vi "MEASURE_hysteresis_multiple_SHG gate_pmt-final - Set voltage_1022D.vi"() -> ()   [LabVIEW 2020]
uses:
  <instrlib>/Keithley 24XX/Public/Data/Read (Multiple Points).vi
  <vilib>/Utility/file.llb/Write Delimited Spreadsheet (DBL).vi
  <instrlib>/Keithley 24XX/Keithley 24XX.lvlib
  <vilib>/Analysis/NI_AALBase.lvlib
panel:
  in  "B Reference Source":u8(ring) items=["External", "Internal", "Internal Sweep"]
  in  "Sample Time (0.01-100s)":u16(ring) items=["62.5 mHz", "125 mHz", "250 mHz", "500 mHz", "1 Hz", "2 Hz", "4 Hz", "8Hz", "16 Hz", "32 Hz", "64 Hz", "128 Hz", "256 Hz", "512 Hz", "Trigger "]
  in  "auto phase B":bool
  in  "B reference Manual Phase":dbl=0.05
  in  "B harmonic 2":u8
  in  "B harmonic 1":u8
  in  "B Sine Output Amplitude":dbl=0.05
  in  "B Input Connection":u16(ring) items=["Single-Ended Voltage", "Differential Voltage", "1 MOhm Current Gain", "100 MOhm Current Gain"]
  in  "B frequency":dbl=50.0 format="%#_13g"
  in  "A Reference Source":u8(ring) items=["External", "Internal", "Internal Sweep"]
  in  "Sample Time (0.01-100s)":u16(ring) items=["62.5 mHz", "125 mHz", "250 mHz", "500 mHz", "1 Hz", "2 Hz", "4 Hz", "8Hz", "16 Hz", "32 Hz", "64 Hz", "128 Hz", "256 Hz", "512 Hz", "Trigger "]
  in  "auto phase A":bool
  in  "A reference Manual Phase":dbl=0.05
  in  "A harmonic 2":u8
  in  "Channel A/B for Parameter1":u8(ring) items=["Channel A", "Channel B"]
  out "top gate leaking":dbl=2.469318360898143e-10
  in  "Parameter1":u16(ring)=1 items=["X", "Y", "R", "Theta", "Frequency", "Noise", "Xh1", "Yh1", "Rh1", "Theta h1", "Xh2", "Yh2", "Rh2", "Theta h2"]
  in  "A harmonic 1":u8
  in  "Set voltage (T)":bool=TRUE
  in  "back Vg final Value":dbl=6.0
  in  "Gate sequence":dbl
  out "while loop":dbl
  in  "bottom gate-off set":dbl=-5.0
  in  "0ff set{T}/no off set[F]":bool
  out "XY Graph 4":cluster{dbl[], sgl[]}(graph)
  out "XY Graph 3":cluster{dbl[], sgl[]}(graph)
  out "back gate leaking":dbl=2.469318360898143e-10
  out "top gate voltage":dbl format="%#_13g"
  in  "Compliance  Level (1uA)":dbl=1.9999999995789155e-07
  in  "Source Mode  (0: Voltage)":u16(ring) items=["Voltage", "Current"]
  in  "Serial Configuration":T1={"Baud Rate"=9600, "Parity"=0, "Data Bits"=8, "Stop Bits"=10, "Flow Control"=0} {"Flow Control" items=["None", "XON/XOFF", "RTS/CTS", "XON/XOFF & RTS/CTS", "DTR/DSR", "XON/XOFF & DTR/DSR"]; "Stop Bits" items=["1.0"=10, "1.5"=15, "2.0"=20]; "Data Bits" items=["7"=7, "8"=8]; "Parity" items=["None", "Odd", "Even", "Mark", "Space"]; "Baud Rate" items=["300"=300, "600"=600, "1200"=1200, "2400"=2400, "4800"=4800, "9600"=9600, "19200"=19200]}
  in  "back gate address":refnum<visa-resource-name>="GPIB0::25::INSTR"
  in  "top gate thickness":dbl=10.0
  in  "back gate thickness":dbl=30.0
  in  "pure field (T)/pure doping (F)":bool
  out "loop run":i32=2
  in  "loop #":i32=2
  in  "Save data or not":bool=TRUE
  in  "path (folder + filename)":string="C:\\Users\\User\\Data\\Jason\\03282019\\ pure_bottom_high_6v_rato3 with light2"
  in  "Clear Plot":bool
  out "LOCKIN Measurement1":dbl=0.9110010000000001
  out "back gate voltage":dbl format="%#_13g"
  in  "GATE STEP(mv)":i32=450
  in  "GATE Low Value (default 0)":dbl
  in  "GATE High Value":dbl=18.0
  in  "Function (0: Volts) 2":u16(ring) items=["Volts", "Current", "Resistance"]
  in  "Source Compaliance":dbl=1.000000000000001e-07
  in  "topgate address":refnum<visa-resource-name>="GPIB0::18::INSTR"
  in  "SD stabilization(S) 2":dbl=0.1 format="%#_13g"
  in  "A Sine Output Amplitude":dbl=0.05
  in  "GATE / SD stablization 3":dbl=0.1 format="%#_13g"
  in  "A Sine output frequency":dbl=50.0 format="%#_13g"
  in  "A Input Connection":u16(ring) items=["Single-Ended Voltage", "Differential Voltage", "1 MOhm Current Gain", "100 MOhm Current Gain"]
  in  "LOCKIN address":refnum<visa-resource-name>="GPIB0::8::INSTR"
  # "Gate2400(Back) Setting"
  # "Lock-in"
  # "Channel A"
  # "Gate2400(Top) Setting"
  # "Channel B"
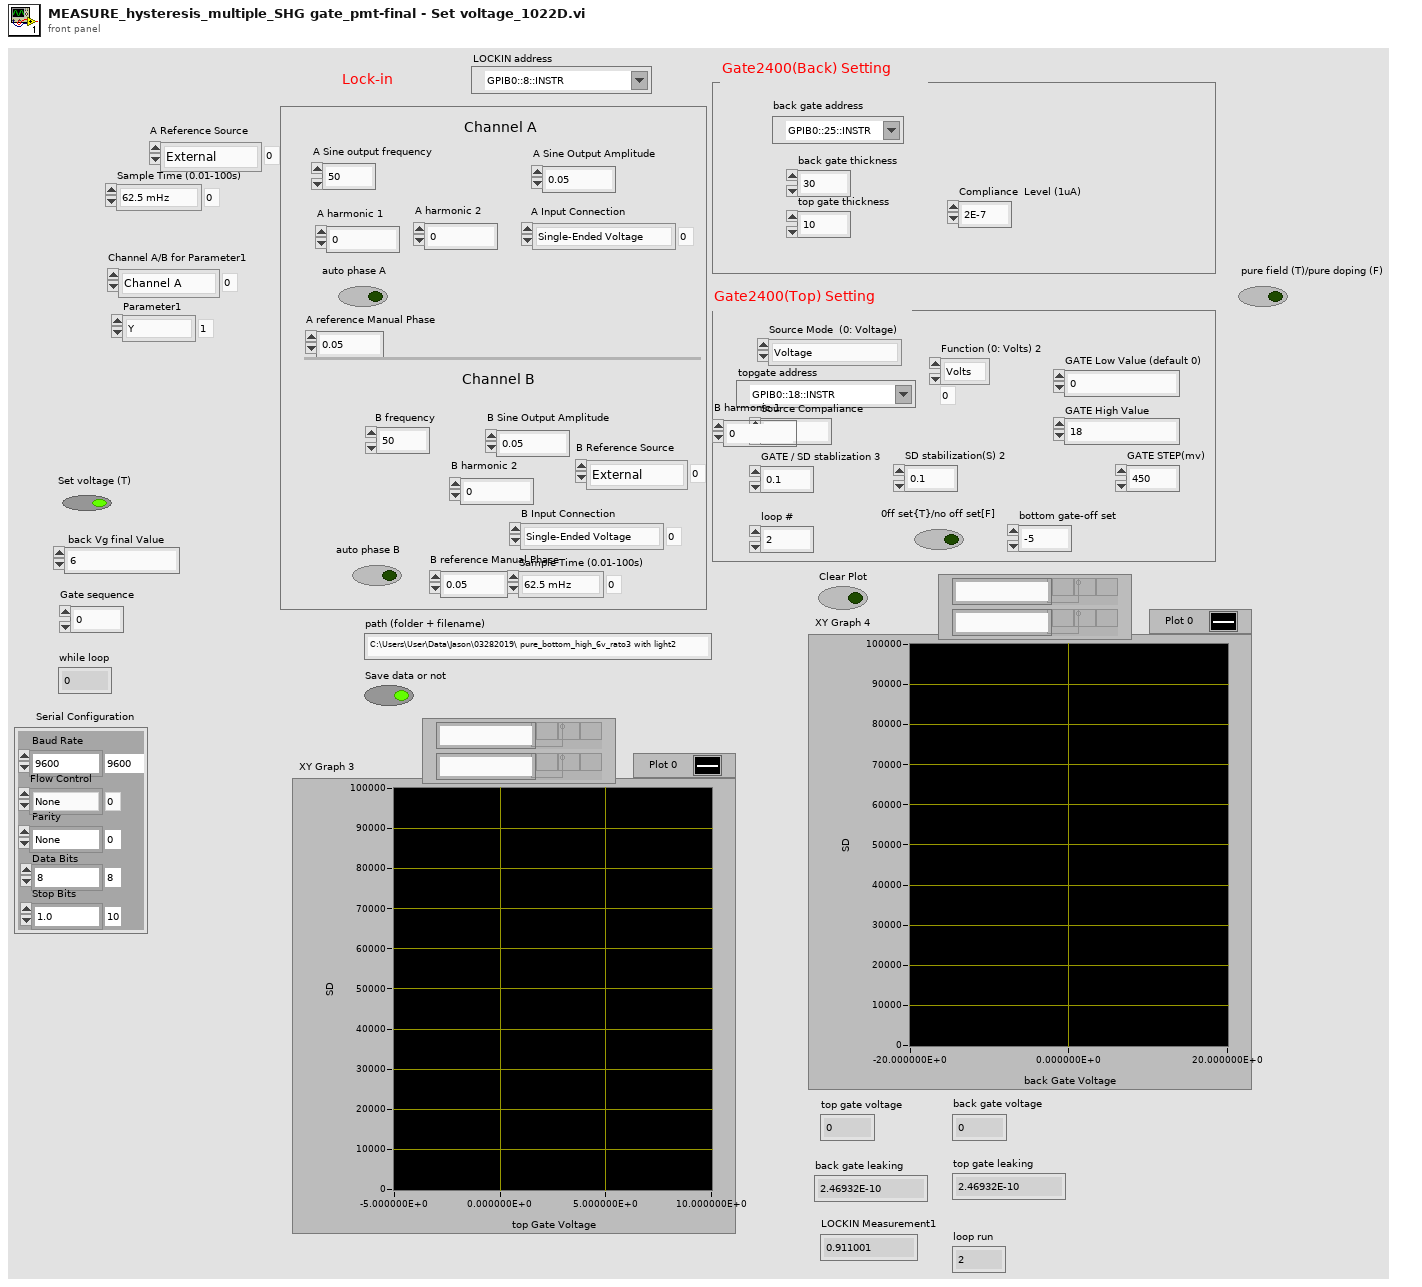
[diagram p1: front panel]
types:
  T1 = cluster{"Baud Rate":u32, "Parity":u16, "Data Bits":u16, "Stop Bits":u16, "Flow Control":u16}
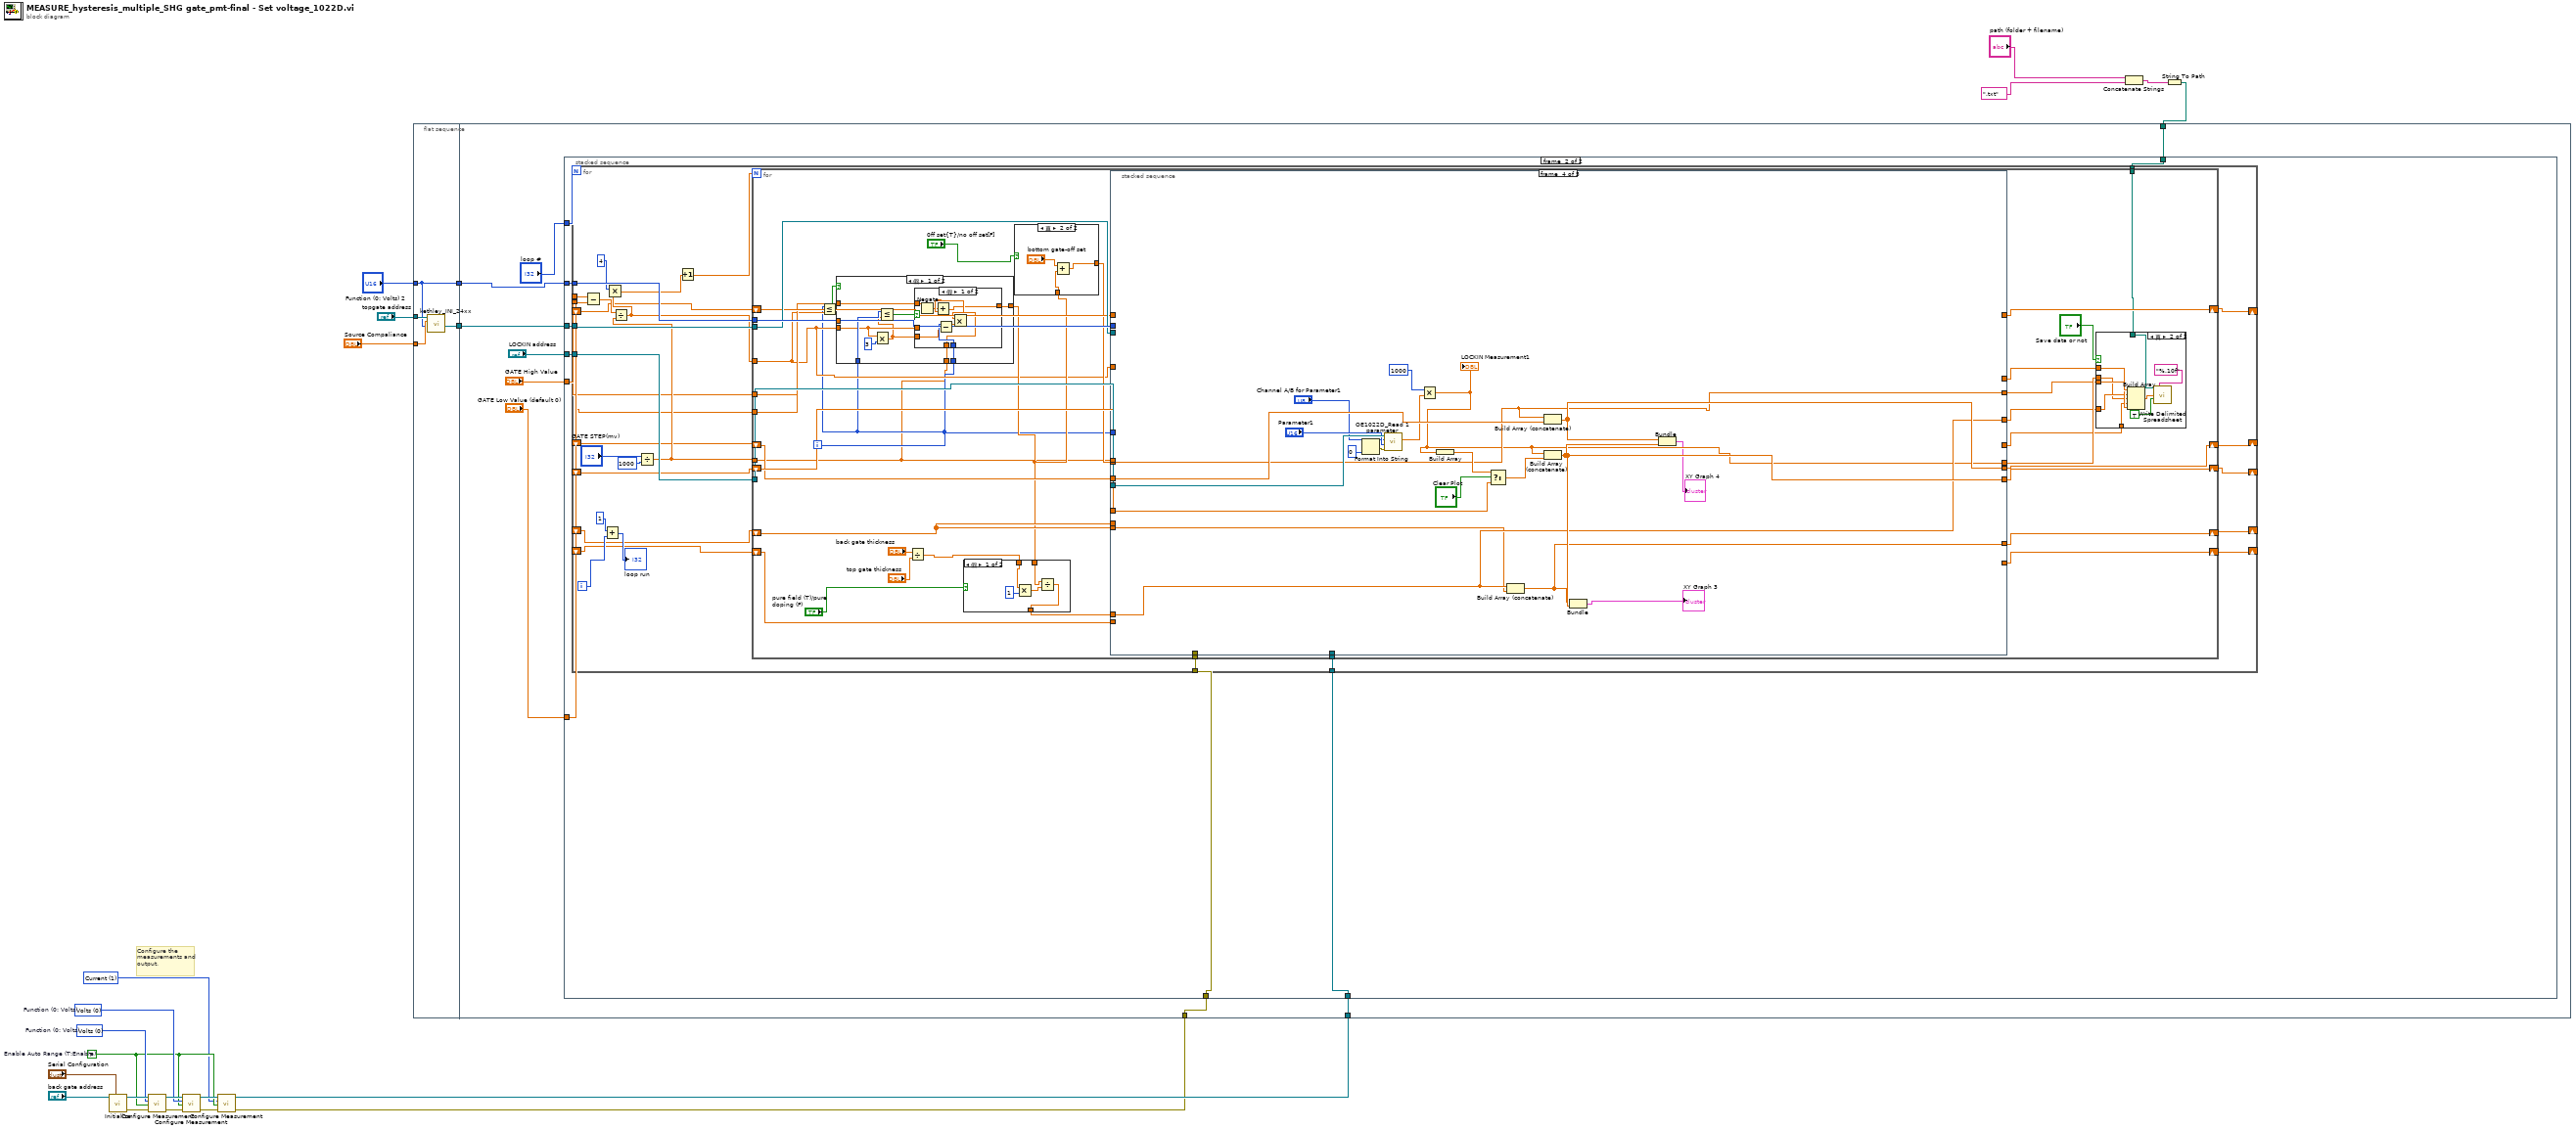
[diagram p0: block diagram]
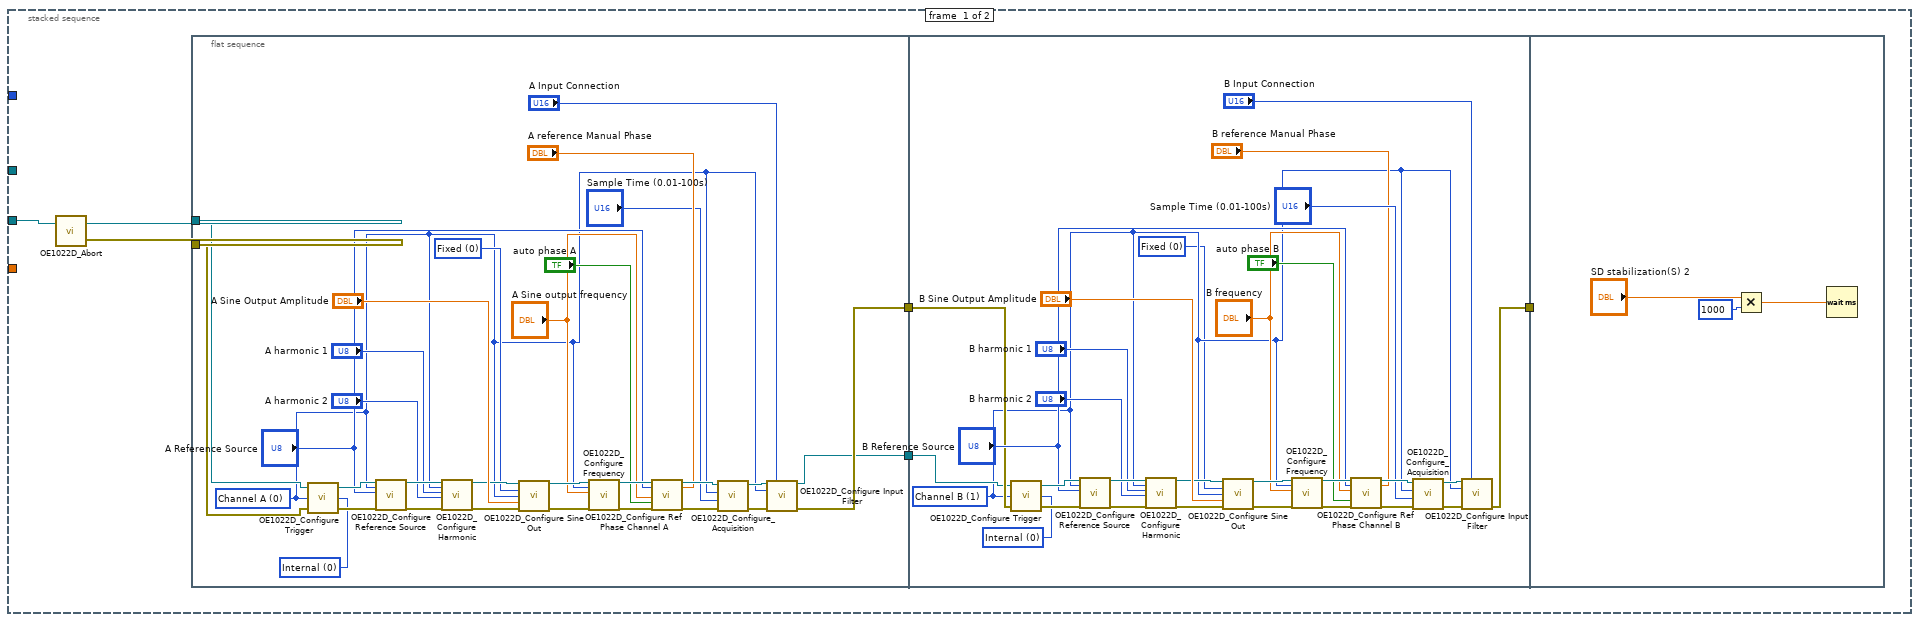
[diagram p2: hidden frame]
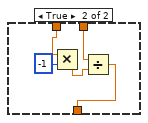
[diagram p4: hidden frame]
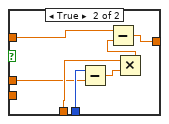
[diagram p6: hidden frame]
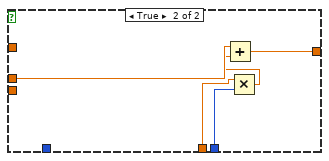
[diagram p7: hidden frame]
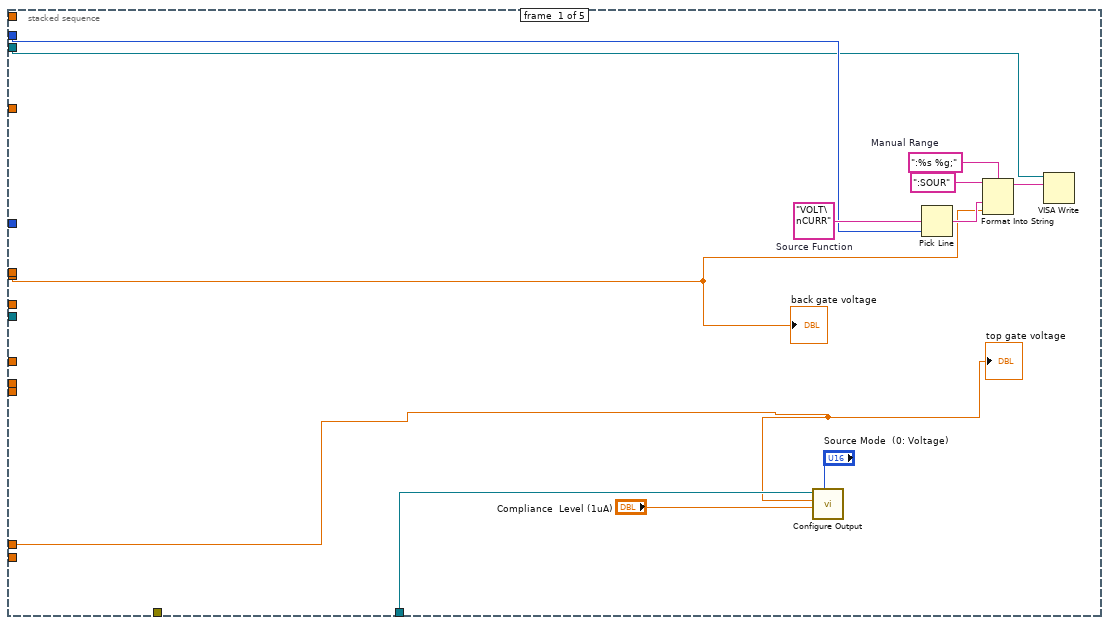
[diagram p8: hidden frame]
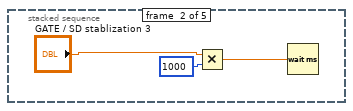
[diagram p9: hidden frame]
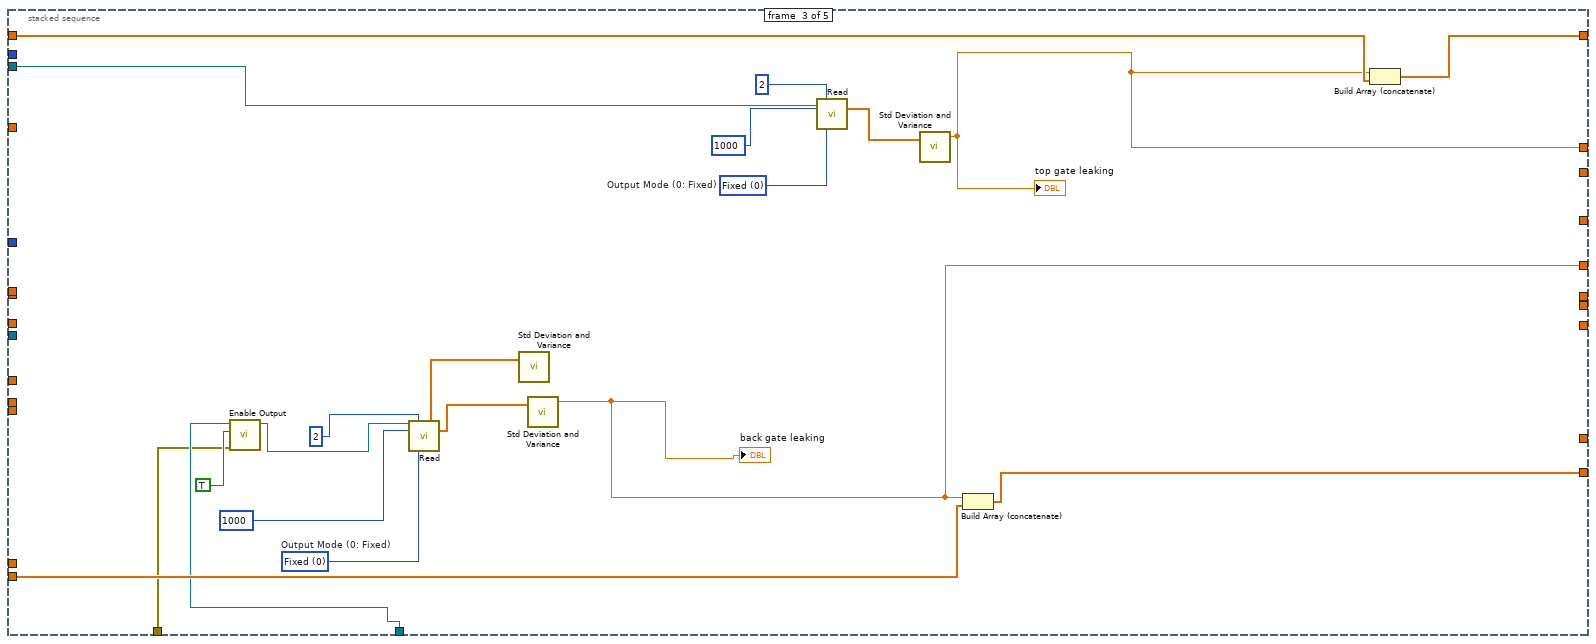
[diagram p10: hidden frame]
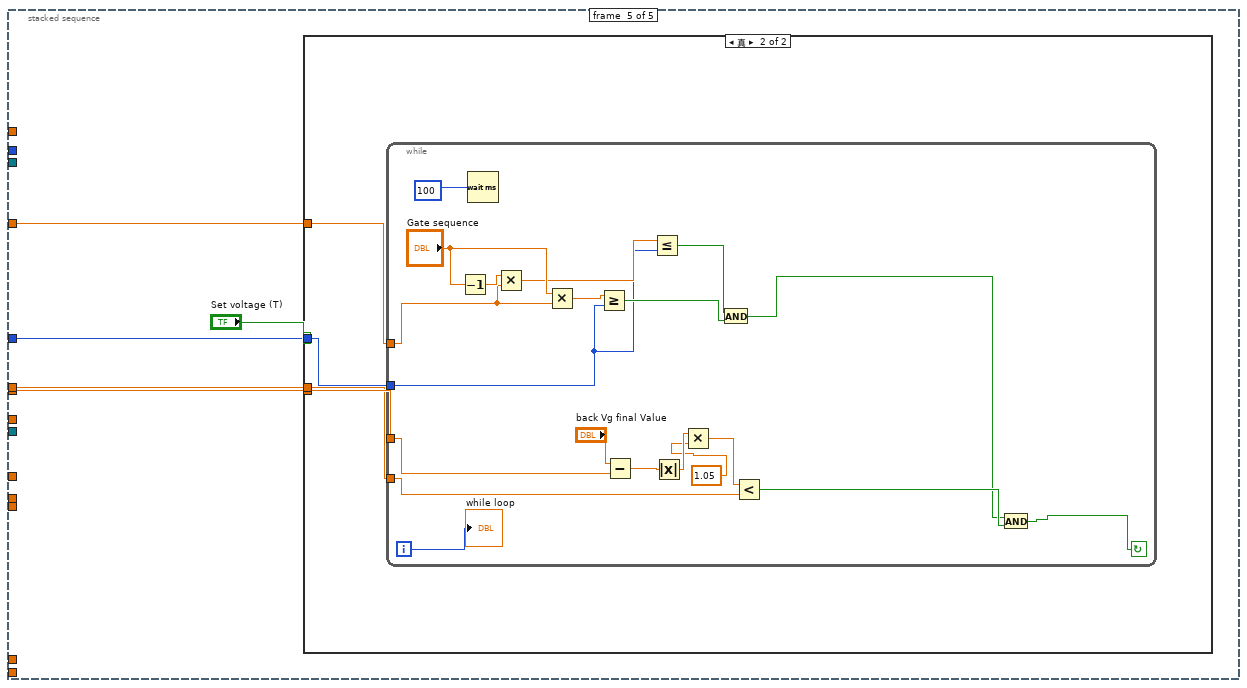
[diagram p11: hidden frame]
diagram:
  w3 = u16 1 items=["Volts", "Current", "Resistance"] ("Function (0: Volts)")
  w4 = TRUE  # Enable Auto Range (T:Enable)
  w7 = u16 0 items=["Volts", "Current", "Resistance"]  # Function (0: Volts)
  w8 = u16 0 items=["Volts", "Current", "Resistance"]  # Function (0: Volts)
  # "Configure the measurements and output."
  n1 = call <instrlib>:"Initialize.vi"("Serial Configuration"="Serial Configuration", "VISA resource name"="back gate address") -> ("error out"=w13:errorcluster, "VISA resource name out"=w14:refnum<visa-resource-name>)  [unwired: 8 in]
  n2 = call <instrlib>:"Configure Measurement.vi"("error in (no error)"=w13, "Enable Auto Range (T:Enable)"=w4, "Function (0: Volts)"=w8, "VISA resource name"=w14) -> ("error out"=w12:errorcluster, "VISA resource name out"=w11:refnum<visa-resource-name>)  [unwired: 6 in]
  n3 = call <instrlib>:"Configure Measurement.vi"("error in (no error)"=w12, "Enable Auto Range (T:Enable)"=w4, "Function (0: Volts)"=w7, "VISA resource name"=w11) -> ("error out"=w5:errorcluster, "VISA resource name out"=w6:refnum<visa-resource-name>)  [unwired: 6 in]
  n4 = call <instrlib>:"Configure Measurement.vi"("error in (no error)"=w5, "Enable Auto Range (T:Enable)"=w4, "Function (0: Volts)"=w3, "VISA resource name"=w6) -> ("error out"=w1:errorcluster, "VISA resource name out"=w2:refnum<visa-resource-name>)  [unwired: 6 in]
  n5 = flat-sequence {
    tunnel: "topgate address" -> [w27]
    tunnel: "Source Compaliance" -> [w26]
    tunnel: "Function (0: Volts) 2" -> [w24]
    tunnel: [w25] -> w20
    tunnel: [w24] -> w19
    tunnel: w20 -> [w35]
    tunnel: w19 -> [w34]
    tunnel: w15 -> [w31]
    tunnel: w2 -> [w29]
    tunnel: w1 -> [w28]
    frame #0 {
      n6 = call "kethley_INI_24xx.vi"("Function (0: Volts) in"=w24, "Source Compaliance"=w26, "VISA Return in"=w27) -> ("VISA resource name out"=w25:refnum<visa-resource-name>)  [unwired: 8 in]
    }
    frame #1 {
      n7 = stacked-sequence {
        tunnel: "LOCKIN address" -> [w42 w111]
        tunnel: w35 -> [_ w112]
        tunnel: w34 -> [_ w113]
        tunnel: "GATE High Value" -> [_ w109]
        tunnel: "GATE Low Value (default 0)" -> [_ w110]
        tunnel: w31 -> [_ w108]
        tunnel: "loop #" -> [_ w107]
        tunnel: w29 -> [_ w106]
        tunnel: w28 -> [_ w105]
        frame #0 {
          n8 = call <instrlib>:"OE1022D_Abort.vi"("VISA resource name"=w42) -> ("error out"=w40:errorcluster, "VISA resource name out"=w41:refnum<visa-resource-name>)  [unwired: 1 in]
          n9 = flat-sequence {
            tunnel: w41 -> [w72]
            tunnel: [w60] -> w39
            tunnel: w40 -> [w71]
            tunnel: [w45] -> w37
            tunnel: w39 -> [w79]
            tunnel: [w78] -> w38
            tunnel: w37 -> [w77]
            tunnel: w38 -> [_]
            frame #0 {
              w44 = u8 0 items=["Fixed", "Linear", "Log"] ("SineOut Mode")
              w46 = u16 0 items=["Internal", "External"] ("Trigger Source (0: Internal)")
              w43 = u8 0 items=["Channel A", "Channel B"] ("OE1022D A/B")
              n10 = call <instrlib>:"OE1022D_Configure Trigger.vi"("Trigger Source (0: Internal)"=w46, "error in (no error)   2"=w71, "OE1022D A/B"=w43, "VISA resource name   2"=w72) -> ("error out   2"=w65:errorcluster, "VISA resource name out   2"=w66:refnum<visa-resource-name>)
              n11 = call <instrlib>:"OE1022D_Configure Reference Source.vi"("VISA resource name"=w66, "OE1022D A/B"=w43, "Reference Source"="A Reference Source", "error in (no error)"=w65) -> ("VISA resource name out"=w64:refnum<visa-resource-name>, "error out"=w62:errorcluster)  [unwired: 14 in]
              n12 = call <instrlib>:"OE1022D_Configure Harmonic.vi"("VISA resource name"=w64, "OE1022D A/B"=w43, "Harmonic 1"="A harmonic 1", "Harmonic 2"="A harmonic 2", "error in (no error)"=w62) -> ("VISA resource name out"=w63:refnum<visa-resource-name>, "error out"=w61:errorcluster)  [unwired: 13 in]
              n13 = call <instrlib>:"OE1022D_Configure Sine Out.vi"("VISA resource name"=w63, "SineOut Mode"=w44, "OE1022D A/B"=w43, "Sine Output Amplitude (V)"="A Sine Output Amplitude", "error in (no error)"=w61) -> ("VISA resource name out"=w69:refnum<visa-resource-name>, "error out"=w68:errorcluster)  [unwired: 9 in]
              n14 = call <instrlib>:"OE1022D_Configure Frequency.vi"("VISA resource name"=w69, "OE1022D A/B"=w43, "Internal Frequency(Hz)"="A Sine output frequency", "error in (no error)"=w68) -> ("VISA resource name out"=w59:refnum<visa-resource-name>, "error out"=w54:errorcluster)  [unwired: 14 in]
              n15 = call <instrlib>:"OE1022D_Configure Ref Phase Channel A.vi"("VISA resource name"=w59, "Reference Source"="A Reference Source", "Internal Frequency(Hz)"="A Sine output frequency", "Auto Phase (T: Enabled)"="auto phase A", "error in (no error)"=w54, "Manual Phase  (degree)"="A reference Manual Phase") -> ("VISA resource name out"=w58:refnum<visa-resource-name>, "error out"=w55:errorcluster)  [unwired: 12 in]
              n16 = call <instrlib>:"OE1022D_Configure_Acquisition.vi"("VISA resource name"=w58, "Channel A/B"=w43, "Sample time (s)"="Sample Time (0.01-100s)", "error in (no error)"=w55) -> ("VISA resource name out"=w57:refnum<visa-resource-name>, "error out"=w56:errorcluster)  [unwired: 5 in]
              n17 = call <instrlib>:"OE1022D_Configure Input Filter.vi"("VISA resource name"=w57, "Input Source"="A Input Connection", "OE1022D A/B"=w43, "error in (no error)"=w56) -> ("VISA resource name out"=w45:refnum<visa-resource-name>, "error out"=w60:errorcluster)  [unwired: 10 in]
            }
            frame #1 {
              w73 = u8 0 items=["Fixed", "Linear", "Log"] ("SineOut Mode")
              w80 = u16 0 items=["Internal", "External"] ("Trigger Source (0: Internal)")
              w74 = u8 1 items=["Channel A", "Channel B"] ("OE1022D A/B")
              n18 = call <instrlib>:"OE1022D_Configure Trigger.vi"("Trigger Source (0: Internal)"=w80, "error in (no error)   2"=w79, "OE1022D A/B"=w74, "VISA resource name   2"=w77) -> ("error out   2"=w96:errorcluster, "VISA resource name out   2"=w97:refnum<visa-resource-name>)
              n19 = call <instrlib>:"OE1022D_Configure Reference Source.vi"("VISA resource name"=w97, "OE1022D A/B"=w74, "Reference Source"="B Reference Source", "error in (no error)"=w96) -> ("VISA resource name out"=w95:refnum<visa-resource-name>, "error out"=w93:errorcluster)  [unwired: 14 in]
              n20 = call <instrlib>:"OE1022D_Configure Harmonic.vi"("VISA resource name"=w95, "OE1022D A/B"=w74, "Harmonic 1"="B harmonic 1", "Harmonic 2"="B harmonic 2", "error in (no error)"=w93) -> ("VISA resource name out"=w94:refnum<visa-resource-name>, "error out"=w92:errorcluster)  [unwired: 13 in]
              n21 = call <instrlib>:"OE1022D_Configure Sine Out.vi"("VISA resource name"=w94, "SineOut Mode"=w73, "OE1022D A/B"=w74, "Sine Output Amplitude (V)"="B Sine Output Amplitude", "error in (no error)"=w92) -> ("VISA resource name out"=w100:refnum<visa-resource-name>, "error out"=w99:errorcluster)  [unwired: 9 in]
              n22 = call <instrlib>:"OE1022D_Configure Frequency.vi"("VISA resource name"=w100, "OE1022D A/B"=w74, "Internal Frequency(Hz)"="B frequency", "error in (no error)"=w99) -> ("VISA resource name out"=w91:refnum<visa-resource-name>, "error out"=w86:errorcluster)  [unwired: 14 in]
              n23 = call <instrlib>:"OE1022D_Configure Ref Phase Channel B.vi"("VISA resource name"=w91, "Reference Source"="B Reference Source", "External Ref Trigger"="B frequency", "Auto Phase (T: Enabled)"="auto phase B", "error in (no error)"=w86, "Manual Phase  (degree)"="B reference Manual Phase") -> ("VISA resource name out"=w90:refnum<visa-resource-name>, "error out"=w87:errorcluster)  [unwired: 12 in]
              n24 = call <instrlib>:"OE1022D_Configure_Acquisition.vi"("VISA resource name"=w90, "Channel A/B"=w74, "Sample time (s)"="Sample Time (0.01-100s)", "error in (no error)"=w87) -> ("VISA resource name out"=w89:refnum<visa-resource-name>, "error out"=w88:errorcluster)  [unwired: 5 in]
              n25 = call <instrlib>:"OE1022D_Configure Input Filter.vi"("VISA resource name"=w89, "Input Source"="B Input Connection", "OE1022D A/B"=w74, "error in (no error)"=w88) -> ("error out"=w78:errorcluster)  [unwired: 10 in, 1 out]
            }
            frame #2 {
              n26 = Multiply(x="SD stabilization(S) 2", y=1000) -> (x*y=w104:dbl)
              n27 = Wait (ms)(milliseconds to wait=w104) -> ()  [unwired: 1 out]
            }
          }
        }
        frame #1 {
          n28 = for {
            N: w107 -> [_]
            tunnel: w113 -> [w142]
            tunnel: w112 -> [w141]
            tunnel: w111 -> [w140]
            tunnel: w110 -> [w134]
            tunnel: w109 -> [w133]
            tunnel: w108 -> [w132]
            shift-right: [w128] -> _
            shift-left: _ -> [w127]
            shift-right: [w126] -> _
            shift-left: _ -> [w124]
            shift-right: [w125] -> _
            shift-left: _ -> [w123]
            shift-right: [w119] -> _
            shift-left: _ -> [w118]
            shift-right: [w117] -> _
            shift-left: _ -> [w116]
            tunnel: w106 -> [w115]
            tunnel: w105 -> [w114]
            i -> [w121]
            n29 = Subtract(x=w133, y=w134) -> (x-y=w136:dbl)
            n30 = Add(x=1, y=w121) -> (x+y=→"loop run":i32)
            n31 = Divide(x="GATE STEP(mv)", y=1000) -> (x/y=w135:dbl)
            n32 = Divide(x=w136, y=w135) -> (x/y=w131:dbl)
            n33 = Multiply(x=4, y=w131) -> (x*y=w130:dbl)
            n34 = Increment(x=w130) -> (x+1=w129:dbl)
            n35 = for {
              N: w129 -> [_]
              tunnel: w142 -> [w178]
              tunnel: w141 -> [w177]
              tunnel: w140 -> [w176]
              tunnel: w135 -> [w144]
              shift-right: [w175] -> w128
              shift-left: w127 -> [w174]
              shift-right: [w171] -> w125
              shift-left: w123 -> [w173]
              shift-right: [w170] -> w126
              shift-left: w124 -> [w172]
              tunnel: w131 -> [w146]
              tunnel: w134 -> [w168]
              tunnel: w133 -> [w167]
              tunnel: w132 -> [w163]
              shift-right: [w161] -> w119
              shift-left: w118 -> [w152]
              shift-right: [w160] -> w117
              shift-left: w116 -> [w151]
              tunnel: w115 -> [w158]
              tunnel: w114 -> [w143]
              i -> [w145]
              n36 = Less Or Equal?(x=w145, y=w146) -> (x <= y?=w169:bool)
              n37 = case shown="假" w169 {
                tunnel: w168 -> [_ w230]
                tunnel: w145 -> [w210 w229]
                tunnel: w144 -> [w209 w228]
                tunnel: [w207 w226] -> w148
                tunnel: w167 -> [w208 _]
                tunnel: w146 -> [w203 _]
                tunnel: w145 -> [w206 _]
                frame False {
                  n38 = Multiply(x=w203, y=3) -> (x*y=w202:dbl)
                  n39 = Less Or Equal?(x=w206, y=w202) -> (x <= y?=w204:bool)
                  n40 = case shown="假" w204 {
                    tunnel: w210 -> [w218 w225]
                    tunnel: w209 -> [w216 w223]
                    tunnel: w208 -> [w212 w221]
                    tunnel: [w214 w220] -> w207
                    tunnel: w203 -> [_ w219]
                    tunnel: w202 -> [w211 _]
                    frame False {
                      n41 = Negate(x=w212) -> (-x=w213:dbl)
                      n42 = Subtract(x=w218, y=w211) -> (x-y=w217:dbl)
                      n43 = Multiply(x=w216, y=w217) -> (x*y=w215:dbl)
                      n44 = Add(x=w213, y=w215) -> (x+y=w214:dbl)
                    }
                    frame True {
                      n45 = Subtract(x=w225, y=w219) -> (x-y=w224:dbl)
                      n46 = Multiply(x=w223, y=w224) -> (x*y=w222:dbl)
                      n47 = Subtract(x=w221, y=w222) -> (x-y=w220:dbl)
                    }
                  }
                }
                frame True {
                  n48 = Multiply(x=w228, y=w229) -> (x*y=w227:dbl)
                  n49 = Add(x=w230, y=w227) -> (x+y=w226:dbl)
                }
              }
              n50 = Divide(x="back gate thickness", y="top gate thickness") -> (x/y=w157:dbl)
              n51 = case shown="假" "pure field (T)/pure doping (F)" {
                tunnel: w157 -> [w186 w192]
                tunnel: [w183 w190] -> w153
                tunnel: w148 -> [w184 w189]
                frame False {
                  n52 = Multiply(x=w186, y=1) -> (x*y=w185:dbl)
                  n53 = Divide(x=w184, y=w185) -> (x/y=w183:dbl)
                }
                frame True {
                  n54 = Multiply(x=w192, y=-1) -> (x*y=w188:dbl)
                  n55 = Divide(x=w189, y=w188) -> (x/y=w190:dbl)
                }
              }
              n56 = case shown="真" "0ff set{T}/no off set[F]" {
                tunnel: w148 -> [w179 w182]
                tunnel: [w179 w180] -> w147
                frame False {
                }
                frame True {
                  n57 = Add(x="bottom gate-off set", y=w182) -> (x+y=w180:dbl)
                }
              }
              n58 = stacked-sequence {
                tunnel: w178 -> [w238 _ _ _ _]
                tunnel: w177 -> [w237 _ w251 _ _]
                tunnel: w176 -> [_ _ _ w279 _]
                tunnel: w147 -> [w236 _ _ w278 w288]
                tunnel: [_ _ w264 _ _] -> w175
                tunnel: w174 -> [_ _ w265 _ _]
                tunnel: w173 -> [_ _ _ w282 _]
                tunnel: w172 -> [_ _ _ w280 _]
                tunnel: [_ _ _ w275 _] -> w171
                tunnel: [_ _ _ w281 _] -> w170
                tunnel: [_ _ _ w270 _] -> w166
                tunnel: [_ _ _ w278 _] -> w165
                tunnel: [_ _ w246 _ _] -> w164
                tunnel: [_ _ w258 _ _] -> w161
                tunnel: [_ _ _ w274 _] -> w160
                tunnel: w151 -> [_ _ _ _ _]
                tunnel: [_ _ _ w273 _] -> w159
                tunnel: [_ _ w257 _ _] -> w150
                tunnel: w158 -> [w234 _ w254 _ _]
                tunnel: w153 -> [w232 _ _ w273 _]
                tunnel: w152 -> [_ _ w256 _ _]
                tunnel: w151 -> [_ _ _ w272 _]
                tunnel: w146 -> [_ _ _ _ w290]
                tunnel: w145 -> [_ _ _ _ w289]
                tunnel: w144 -> [_ _ _ _ w287]
                tunnel: w143 -> [_ _ w252 _ _]
                frame #0 {
                  w240 = "VOLT\nCURR"  # Source Function
                  w241 = ":%s %g;"  # Manual Range
                  n59 = call <instrlib>:"Configure Output.vi"("Source Mode  (0: Voltage)"="Source Mode  (0: Voltage)", "Compliance  Level (0.1)"="Compliance  Level (1uA)", "Output Level (0)"=w232, "VISA resource name"=w234) -> ()  [unwired: 6 in, 2 out]
                  n60 = Pick Line(multi-line string=w240, line index=w238) -> (output string=w239:string)  [unwired: 1 out]
                  n61 = Format Into String(format string=w241, initial string=":SOUR" ("Manual Range"), w239, w236) -> (resulting string=w242:string)  [unwired: 1 in, 1 out]
                  n62 = VISA Write(VISA resource name=w237, write buffer=w242) -> ()  [unwired: 1 in, 3 out]
                  "back gate voltage" <- w236
                  "top gate voltage" <- w232
                }
                frame #1 {
                  n63 = Multiply(x="GATE / SD stablization 3", y=1000) -> (x*y=w245:dbl)
                  n64 = Wait (ms)(milliseconds to wait=w245) -> ()  [unwired: 1 out]
                }
                frame #2 {
                  w247 = u16 0 items=["Fixed", "Sweep", "List"]  # Output Mode (0: Fixed)
                  w261 = u16 0 items=["Fixed", "Sweep", "List"]  # Output Mode (0: Fixed)
                  n65 = call <instrlib>:"Enable Output.vi"("error in (no error)"=w252, "Enable Output (T: Enable)"=TRUE, "VISA resource name"=w254) -> ("VISA resource name out"=w253:refnum<visa-resource-name>)  [unwired: 7 in, 1 out]
                  n66 = call-poly <instrlib>:"Read.vi"("VISA resource name"=w253, "Sample Count (1)"=u32 2 ("Number of Samples"), "Timeout (10000 ms)"=1000, "Output Mode (0: Fixed)"=w261) -> ("Voltage"=w259:sgl[], "Current"=w260:sgl[])  [unwired: 5 in, 5 out]
                  n67 = call <vilib>:"Std Deviation and Variance.vi"("X"=w259) -> ()  [unwired: 1 in, 3 out]
                  n68 = call <vilib>:"Std Deviation and Variance.vi"("X"=w260) -> ("mean"=w257:dbl)  [unwired: 1 in, 2 out]
                  "back gate leaking" <- w257
                  n69 = call-poly <instrlib>:"Read.vi"("VISA resource name"=w251, "Sample Count (1)"=u32 2 ("Number of Samples"), "Timeout (10000 ms)"=1000, "Output Mode (0: Fixed)"=w247) -> ("Current"=w250:sgl[])  [unwired: 5 in, 6 out]
                  n70 = call <vilib>:"Std Deviation and Variance.vi"("X"=w250) -> ("mean"=w246:dbl)  [unwired: 1 in, 2 out]
                  "top gate leaking" <- w246
                  n71 = Build Array (concatenate)(w257, w256) -> (w258:dbl[])
                  n72 = Build Array (concatenate)(w246, w265) -> (w264:dbl[])
                }
                frame #3 {
                  n73 = Format Into String(0) -> (error out=w286:errorcluster)  [unwired: 3 in, 1 out]
                  n74 = call <instrlib>:"OE1022D_Read 1 parameter.vi"("错误输入（无错误）"=w286, "Parameter"="Parameter1", "Channel (0: A)"="Channel A/B for Parameter1", "VISA resource name"=w279) -> ("Measurement"=w267:sgl)  [unwired: 5 in, 2 out]
                  n75 = Multiply(x=1000, y=w267) -> (x*y=w270:sgl)
                  "LOCKIN Measurement1" <- w270
                  n76 = Build Array(w270) -> (w284:sgl[])
                  n77 = Select(t=w284, s="Clear Plot", f=w282) -> (s? t:f=w277:sgl[])
                  n78 = Build Array (concatenate)(w273, w272) -> (w274:dbl[])
                  n79 = Build Array (concatenate)(w278, w280) -> (w281:dbl[])
                  n80 = Build Array (concatenate)(w270, w277) -> (w275:sgl[])
                  n81 = Bundle(w274, w275) -> (→"XY Graph 3":cluster{dbl[], sgl[]})  [unwired: 1 in]
                  n82 = Bundle(w281, w275) -> (→"XY Graph 4":cluster{dbl[], sgl[]})  [unwired: 1 in]
                }
                frame #4 {
                  n83 = case shown="真" "Set voltage (T)" {
                    tunnel: w290 -> [_ w295]
                    tunnel: w289 -> [_ w294]
                    tunnel: w288 -> [_ w293]
                    tunnel: w287 -> [_ w292]
                    frame False {
                    }
                    frame True {
                      n84 = while {
                        tunnel: w294 -> [w301]
                        tunnel: w295 -> [w305]
                        tunnel: w292 -> [w310]
                        tunnel: w293 -> [w308]
                        i -> [w315]
                        stop <- w313 continue-if-true
                        n85 = Decrement(x="Gate sequence") -> (x-1=w306:dbl)
                        n86 = Wait (ms)(milliseconds to wait=100) -> ()  [unwired: 1 out]
                        n87 = Multiply(x=w306, y=w305) -> (x*y=w302:dbl)
                        n88 = Multiply(x="Gate sequence", y=w305) -> (x*y=w304:dbl)
                        n89 = Greater Or Equal?(x=w304, y=w301) -> (x >= y?=w303:bool)
                        n90 = Subtract(x="back Vg final Value", y=w308) -> (x-y=w311:dbl)
                        n91 = Less Or Equal?(x=w302, y=w301) -> (x <= y?=w300:bool)
                        n92 = Absolute Value(x=w311) -> (abs(x)=w298:dbl)
                        n93 = Multiply(x=w298, y=1.05) -> (x*y=w297:dbl)
                        n94 = And(x=w300, y=w303) -> (x .and. y?=w299:bool)
                        n95 = Less?(x=w297, y=w310) -> (x < y?=w309:bool)
                        n96 = And(x=w299, y=w309) -> (x .and. y?=w313:bool)
                        "while loop" <- w315
                      }
                    }
                  }
                }
              }
              n97 = case shown="真" "Save data or not" {
                tunnel: w166 -> [_ w194]
                tunnel: w165 -> [_ w201]
                tunnel: w164 -> [_ w200]
                tunnel: w163 -> [_ w198]
                tunnel: w159 -> [_ w195]
                tunnel: w150 -> [_ w193]
                frame False {
                }
                frame True {
                  n98 = Build Array(w201, w195, w194, w193, w200) -> (w199:dbl[])
                  n99 = call-poly <vilib>:"Write Delimited Spreadsheet.vi"("file path (dialog if empty)"=w198, "format (%.3f)"="%.10f", "1D data"=w199, "append to file? (new file:F)"=TRUE) -> ()  [unwired: 10 in, 2 out]
                }
              }
            }
          }
        }
      }
    }
  }
  n100 = Concatenate Strings("path (folder + filename)", ".txt") -> (w16:string)
  n101 = String To Path(string=w16) -> (path=w15:path)
